vi "Raycaster_DrawSprites.vi"(9 "Decorations In":T6, 10 "Game State":T2, 11 "Frame Buffers In":T1) -> (3 "Frame Buffers Out":T1)   [LabVIEW 2020]
uses:
  Controls/Raycaster_DrawState.ctl
  Controls/Map_Objects.ctl
  Controls/Map_Object.ctl
  Controls/Map_Position.ctl
  Controls/Game_State.ctl
  Controls/Player_LocationInfo.ctl
  Controls/Player_LocationInfoAxis.ctl
  Math_Subtract_FXP.vi
  Math_Reciprocal.vi
  Globals/MAX_SPRITES.vi
  Globals/WIDTH_DIV_2.vi
  Globals/WIDTH.vi
  Globals/HEIGHT_DIV_2.vi
  Sprite_GetSprites.vi
  <vilib>/Utility/file.llb/Application Directory.vi
  <vilib>/picture/bmp.llb/Read BMP File.vi
  <vilib>/rvi/DataTransferAndStorage/Container/XNode/niFpgaContainer.xnode
  <vilib>/rvi/DataTransferAndStorage/Register/Emulation/niFpgaRegisterEmulation.vi
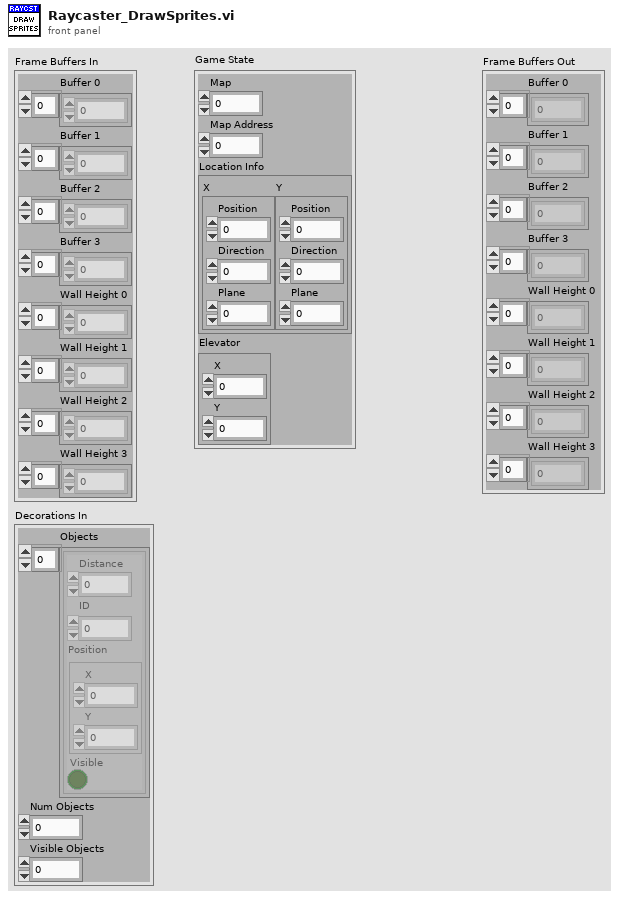
[diagram p1: front panel]
types:
  T1 = typedef "Raycaster_DrawState.ctl" = cluster{"Buffer 0":u8[], "Buffer 1":u8[], "Buffer 2":u8[], "Buffer 3":u8[], "Wall Height 0":i16[], "Wall Height 1":i16[], "Wall Height 2":i16[], "Wall Height 3":i16[]}
  T2 = typedef "Game_State.ctl" = cluster{"Map":u8, "Map Address":u32, "Location Info":T3, "Elevator":T5}
  T3 = typedef "Player_LocationInfo.ctl" = cluster{"X":T4, "Y":T4}
  T4 = typedef "Player_LocationInfoAxis.ctl" = cluster{"Position":fxp<+/-,32,16>, "Direction":fxp<+/-,32,16>, "Plane":fxp<+/-,32,16>}
  T5 = typedef "Map_Position.ctl" = cluster{"X":fxp<+/-,32,16>, "Y":fxp<+/-,32,16>}
  T6 = typedef "Map_Objects.ctl" = cluster{"Objects":T7[], "Num Objects":i16, "Visible Objects":i16}
  T7 = typedef "Map_Object.ctl" = cluster{"Distance":fxp<+/-,32,16>, "ID":u8, "Position":T5, "Visible":bool}
  T8 = typedef "Raycaster_ScreenCalcs.ctl" = cluster{"Length":i16, "Pixel Start":i16, "Pixel End":i16, "Draw Start":i16}
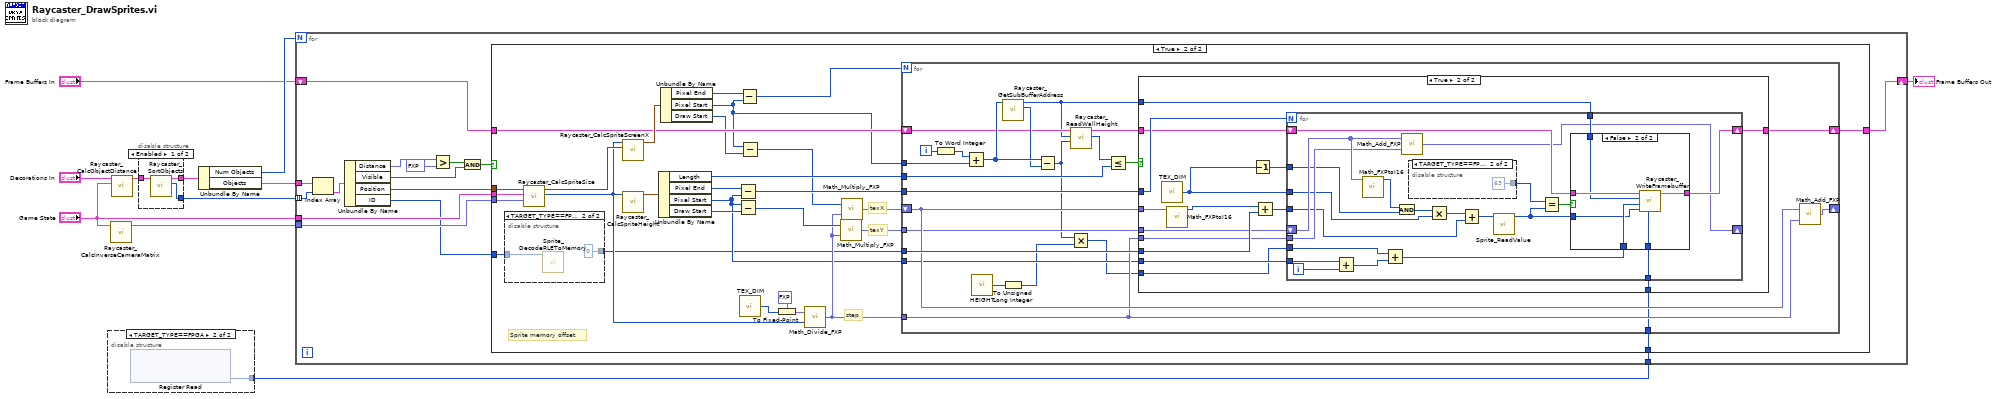
[diagram p0: block diagram]
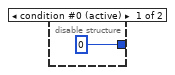
[diagram p2: hidden frame]
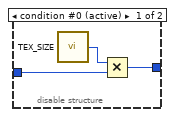
[diagram p5: hidden frame]
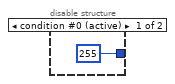
[diagram p7: hidden frame]
diagram:
  n1 = disable-structure "Conditional Disable Structure" shown="TARGET_TYPE==FPGA" {
    disable-tunnel: [u8 0 ("Data") w13] -> w5
    frame condition #0 (active) {
    }
    frame condition #1 {
      n2 = xnode ("Register Read")() -> ("Data"=w13:u8)  [unwired: 1 in, 1 out]
    }
  }
  n3 = call "Raycaster_CalcInverseCameraMatrix.vi"("Location Info"="Game State") -> ("Inverse Matrix"=w7:fxp<+/-,32,16>)  [unwired: 10 in]
  n4 = call "Raycaster_CalcObjectDistance.vi"("Location Info"="Game State", "Decorations In"="Decorations In") -> ("Decorations Out"=w9:T6)  [unwired: 9 in]
  n5 = disable-structure shown="Enabled" {
    disable-tunnel: w9 -> [w16 w17]
    disable-tunnel: [w15 w17] -> w8
    disable-tunnel: [w14 _] -> w6
    frame Enabled {
      n6 = call "Raycaster_SortObjects.vi"("Decorations In"=w16) -> ("Sorted Indexes"=w14:u8[], "Decorations Out"=w15:T6)  [unwired: 9 in]
    }
    frame Disabled {
    }
  }
  n7 = Unbundle By Name(w8) -> ("Num Objects"=w11:i16, "Objects"=w10:T7[])
  n8 = for {
    N: w11 -> [_]
    tunnel: w10 -> [w30]
    shift-right: [w32] -> w1
    shift-left: "Frame Buffers In" -> [w31]
    tunnel: w7 -> [w22]
    tunnel: "Game State" -> [w23]
    tunnel: w6 -> [w19] mode=indexing
    tunnel: w5 -> [w18]
    n9 = Index Array(array=w30, index=w19) -> (element=w20:T7)
    n10 = Unbundle By Name(w20) -> ("Distance"=w29:fxp<+/-,32,16>, "Visible"=w26:bool, "Position"=w24:T5, "ID"=w21:u8)
    n11 = Greater?(x=w29, y=fxp<+/-,32,16> 0.25) -> (0:w27:bool)
    n12 = And(x=w27, y=w26) -> (x .and. y?=w25:bool)
    n13 = case shown="True" w25 {
      tunnel: w23 -> [_ w57]
      tunnel: w31 -> [w33 w54]
      tunnel: [w33 w53] -> w32
      tunnel: w24 -> [_ w58]
      tunnel: w22 -> [_ w50]
      tunnel: w21 -> [_ w36]
      tunnel: w18 -> [_ w34]
      frame False {
      }
      frame True {
        # "Sprite memory offset"
        # "texX"
        # "step"
        # "texY"
        n14 = disable-structure shown="TARGET_TYPE==FPGA" {
          disable-tunnel: w36 -> [w64 w67]
          disable-tunnel: [w63 u32 0] -> w35
          frame condition #0 (active) {
            n15 = call "TEX_SIZE.vi"() -> ("TEX_SIZE"=w65:u32)
            n16 = Multiply(x=w65, y=w64) -> (x*y=w63:u32)
          }
          frame condition #1 {
            n17 = call "Sprite_DecodeRLEToMemory.vi"("Sprite ID"=w67) -> ()  [unwired: 11 in]
          }
        }
        n18 = call "Raycaster_CalcSpriteSize.vi"("Inverse Matrix"=w50, "Location Info"=w57, "Object Position"=w58) -> ("Sprite Size"=w47:i16, "Sprite X Position"=w56:i16)  [unwired: 7 in]
        n19 = call "Raycaster_CalcSpriteScreenX.vi"("Sprite Screen X"=w56, "Object Width"=w47) -> ("Width Calcs"=w62:T8)  [unwired: 9 in]
        n20 = call "Raycaster_CalcSpriteHeight.vi"("Object Height"=w47) -> ("Height Calcs"=w60:T8)  [unwired: 10 in]
        n21 = Unbundle By Name(w60) -> ("Length"=w52:i16, "Pixel End"=w59:i16, "Pixel Start"=w37:i16, "Draw Start"=w43:i16)
        n22 = Unbundle By Name(w62) -> ("Pixel End"=w61:i16, "Pixel Start"=w46:i16, "Draw Start"=w42:i16)
        n23 = Subtract(x=w59, y=w37) -> (x-y=w51:i16)
        n24 = Subtract(x=w37, y=w43) -> (x-y=w44:i16)
        n25 = Subtract(x=w61, y=w46) -> (x-y=w55:i16)
        n26 = Subtract(x=w46, y=w42) -> (x-y=w45:i16)
        n27 = call "TEX_DIM.vi"() -> ("TEX_DIM"=w38:i16)
        n28 = To Fixed-Point(fixed-point type=fxp<+/-,32,16> 0.0, number=w38) -> (fixed-point=w49:fxp<+/-,32,16>)
        n29 = call "Math_Divide_FXP.vi"("y"=w47, "x"=w49) -> ("x*y"=w41:fxp<+/-,32,16>)
        n30 = call "Math_Multiply_FXP.vi"("y"=w41, "x"=w44) -> ("x*y"=w39:fxp<+/-,32,16>)
        n31 = call "Math_Multiply_FXP.vi"("y"=w41, "x"=w45) -> ("x*y"=w40:fxp<+/-,32,16>)
        n32 = for {
          N: w55 -> [_]
          shift-right: [w80] -> w53
          shift-left: w54 -> [w70]
          tunnel: w52 -> [w88]
          tunnel: w46 -> [w91]
          tunnel: w51 -> [w81]
          tunnel: w35 -> [w85]
          tunnel: w41 -> [w82]
          tunnel: w39 -> [w83]
          shift-right: [w86] -> _
          shift-left: w40 -> [w84]
          tunnel: w37 -> [w79]
          tunnel: w34 -> [w73]
          i -> [w90]
          n33 = To Word Integer(number=w90) -> (16bit integer=w89:i16)
          n34 = Add(x=w89, y=w91) -> (x+y=w75:i16)
          n35 = call "HEIGHT.vi"() -> ("HEIGHT"=w78:i16)
          n36 = call "Raycaster_GetSubBufferAddress.vi"("Column"=w75) -> ("Start Address"=w74:i16, "Sub Buffer"=w68:u8)  [unwired: 9 in]
          n37 = To Unsigned Long Integer(number=w78) -> (unsigned 32bit integer=w77:u32)
          n38 = Subtract(x=w75, y=w74) -> (x-y=w72:i16)
          n39 = call "Raycaster_ReadWallHeight.vi"("Sub Buffer Address"=w72, "Sub Buffer"=w68, "Frame Buffers In"=w70) -> ("Height"=w71:i16, "Frame Buffers Out"=w69:T1)  [unwired: 7 in]
          n40 = Multiply(x=w72, y=w77) -> (x*y=w76:u32)
          n41 = Less Or Equal?(x=w71, y=w88) -> (x <= y?=w87:bool)
          n42 = case shown="True" w87 {
            tunnel: w84 -> [_ w97]
            tunnel: w85 -> [_ w107]
            tunnel: w83 -> [_ w106]
            tunnel: w82 -> [_ w105]
            tunnel: w81 -> [_ w104]
            tunnel: w69 -> [w92 w103]
            tunnel: [w92 w102] -> w80
            tunnel: w79 -> [_ w99]
            tunnel: w76 -> [_ w98]
            tunnel: w68 -> [_ w94]
            tunnel: w73 -> [_ w93]
            frame False {
            }
            frame True {
              n43 = call "TEX_DIM.vi"() -> ("TEX_DIM"=w96:i16)
              n44 = call "Math_FXPtoI16.vi"("FXP"=w97) -> ("I16"=w95:i16)  [unwired: 10 in]
              n45 = Decrement(x=w96) -> (x-1=w101:i16)
              n46 = Add(x=w95, y=w107) -> (x+y=w100:u32)
              n47 = for {
                N: w104 -> [_]
                shift-right: [w108] -> _
                shift-left: w106 -> [w128]
                tunnel: w105 -> [w127]
                shift-right: [w122] -> w102
                shift-left: w103 -> [w123]
                tunnel: w101 -> [w126]
                tunnel: w100 -> [w125]
                tunnel: w99 -> [w121]
                tunnel: w98 -> [w119]
                tunnel: w96 -> [w114]
                tunnel: w94 -> [w113]
                tunnel: w93 -> [w109]
                i -> [w120]
                n48 = Add(x=w121, y=w120) -> (x+y=w118:i32)
                n49 = call "Math_FXPtoI16.vi"("FXP"=w128) -> ("I16"=w129:i16)  [unwired: 10 in]
                n50 = Add(x=w119, y=w118) -> (x+y=w117:u32)
                n51 = And(x=w129, y=w126) -> (x .and. y?=w116:i16)
                n52 = call "Math_Add_FXP.vi"("y"=w127, "x"=w128) -> ("x*y"=w108:fxp<+/-,32,16>)
                n53 = disable-structure shown="TARGET_TYPE==FPGA" {
                  disable-tunnel: [u8 255 u8 63] -> w112
                  frame condition #0 (active) {
                  }
                  frame condition #1 {
                  }
                }
                n54 = Multiply(x=w116, y=w114) -> (x*y=w115:i16)
                n55 = Add(x=w115, y=w125) -> (x+y=w124:u32)
                n56 = call "Sprite_ReadValue.vi"("Address"=w124) -> ("Value"=w110:u8)  [unwired: 10 in]
                n57 = Equal?(x=w112, y=w110) -> (x = y?=w111:bool)
                n58 = case shown="False" w111 {
                  tunnel: w123 -> [w132 w138]
                  tunnel: [w132 w136] -> w122
                  tunnel: w117 -> [_ w134]
                  tunnel: w113 -> [_ w137]
                  tunnel: w110 -> [_ w133]
                  tunnel: w109 -> [_ w135]
                  frame True {
                  }
                  frame False {
                    n59 = call "Raycaster_WriteFramebuffer.vi"("Offscreen Buffer"=w135, "Value"=w133, "Sub Buffer Address"=w134, "Sub Buffer"=w137, "Frame Buffers In"=w138) -> ("Frame Buffers Out"=w136:T1)  [unwired: 6 in]
                  }
                }
              }
            }
          }
          n60 = call "Math_Add_FXP.vi"("y"=w82, "x"=w84) -> ("x*y"=w86:fxp<+/-,32,16>)
        }
      }
    }
  }
  "Frame Buffers Out" <- w1
